vi "check_point_inside_rect.vi"(5 "rectangle corner":dbl[][](array[numeric]), 8 "Y":dbl[](array[numeric]), 11 "X":dbl[](array[numeric])) -> (3 "result":bool)   [LabVIEW 2017]
panel:
  out "py":dbl
  out "px":dbl
  out "p4y":dbl
  out "p4x":dbl
  out "p3y":dbl
  out "p3x":dbl
  out "p2y":dbl
  out "p2x":dbl
  out "p1y":dbl
  out "p1x":dbl
  out "length condition":bool
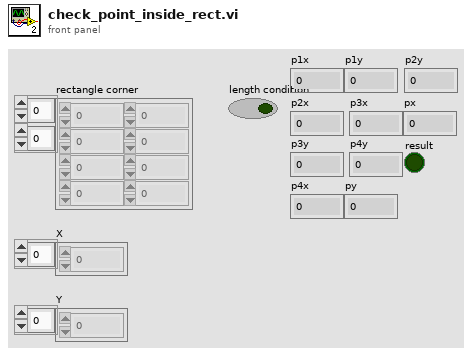
[diagram p1: front panel]
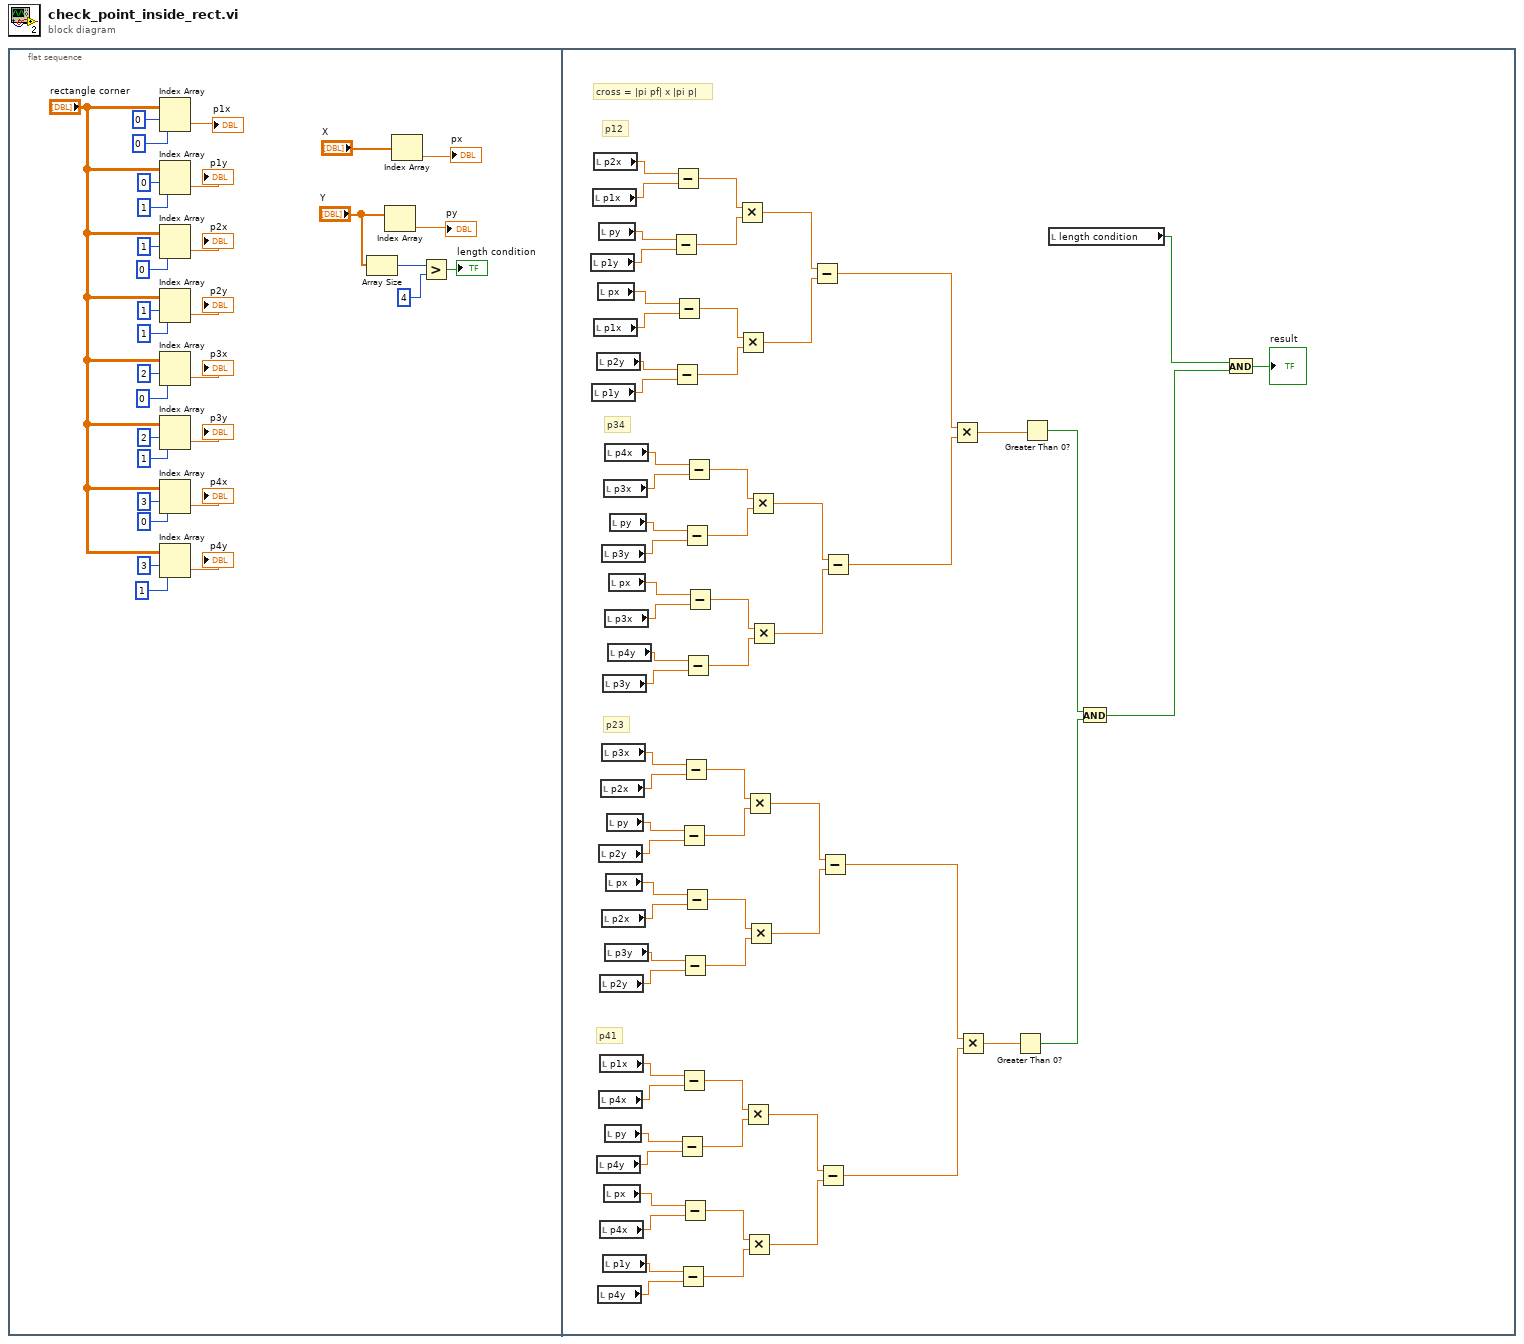
[diagram p0: block diagram]
diagram:
  n1 = flat-sequence {
    frame #0 {
      n2 = Index Array(array="rectangle corner", index (row)=0, index (col)=0 ("disabled index (col)")) -> (element=→"p1x":dbl)
      n3 = Index Array(array="rectangle corner", index (row)=0, index (col)=1 ("disabled index (col)")) -> (element=→"p1y":dbl)
      n4 = Index Array(array="rectangle corner", index (row)=1, index (col)=0 ("disabled index (col)")) -> (element=→"p2x":dbl)
      n5 = Index Array(array="rectangle corner", index (row)=1, index (col)=1 ("disabled index (col)")) -> (element=→"p2y":dbl)
      n6 = Index Array(array="rectangle corner", index (row)=2, index (col)=0 ("disabled index (col)")) -> (element=→"p3x":dbl)
      n7 = Index Array(array="rectangle corner", index (row)=2, index (col)=1 ("disabled index (col)")) -> (element=→"p3y":dbl)
      n8 = Index Array(array="rectangle corner", index (row)=3, index (col)=0 ("disabled index (col)")) -> (element=→"p4x":dbl)
      n9 = Index Array(array="rectangle corner", index (row)=3, index (col)=1 ("disabled index (col)")) -> (element=→"p4y":dbl)
      n10 = Array Size(array="Y") -> (size(s)=w4:i32)
      n11 = Index Array(array="Y") -> (element=→"py":dbl)  [unwired: 1 in]
      n12 = Index Array(array="X") -> (element=→"px":dbl)  [unwired: 1 in]
      n13 = Greater?(x=w4, y=4) -> (0:→"length condition":bool)
    }
    frame #1 {
      # "p41"
      # "p34"
      # "p23"
      # "cross = |pi pf| x |pi p|"
      # "p12"
      n14 = local read "p1y"() -> (w96:dbl)
      n15 = local read "p1y"() -> (w91:dbl)
      n16 = local read "p1x"() -> (w98:dbl)
      n17 = local read "p2x"() -> (w99:dbl)
      n18 = local read "p1x"() -> (w89:dbl)
      n19 = local read "p2y"() -> (w90:dbl)
      n20 = local read "p4y"() -> (w47:dbl)
      n21 = local read "px"() -> (w88:dbl)
      n22 = local read "p4y"() -> (w52:dbl)
      n23 = local read "py"() -> (w97:dbl)
      n24 = local read "p2y"() -> (w75:dbl)
      n25 = local read "p4x"() -> (w45:dbl)
      n26 = local read "p2y"() -> (w80:dbl)
      n27 = local read "p1x"() -> (w44:dbl)
      n28 = local read "p4x"() -> (w54:dbl)
      n29 = local read "p2x"() -> (w73:dbl)
      n30 = local read "p3y"() -> (w68:dbl)
      n31 = local read "p3x"() -> (w72:dbl)
      n32 = local read "p2x"() -> (w82:dbl)
      n33 = local read "p3y"() -> (w63:dbl)
      n34 = local read "p1y"() -> (w53:dbl)
      n35 = local read "p3x"() -> (w70:dbl)
      n36 = local read "px"() -> (w55:dbl)
      n37 = local read "p4x"() -> (w71:dbl)
      n38 = local read "p3x"() -> (w61:dbl)
      n39 = local read "p3y"() -> (w81:dbl)
      n40 = local read "py"() -> (w46:dbl)
      n41 = local read "px"() -> (w83:dbl)
      n42 = local read "py"() -> (w74:dbl)
      n43 = local read "p4y"() -> (w62:dbl)
      n44 = local read "px"() -> (w60:dbl)
      n45 = local read "py"() -> (w69:dbl)
      n46 = Subtract(x=w97, y=w96) -> (x-y=w94:dbl)
      n47 = Subtract(x=w90, y=w91) -> (x-y=w93:dbl)
      n48 = Subtract(x=w99, y=w98) -> (x-y=w95:dbl)
      n49 = Subtract(x=w88, y=w89) -> (x-y=w92:dbl)
      n50 = Subtract(x=w46, y=w47) -> (x-y=w49:dbl)
      n51 = Subtract(x=w53, y=w52) -> (x-y=w50:dbl)
      n52 = Subtract(x=w74, y=w75) -> (x-y=w77:dbl)
      n53 = Subtract(x=w44, y=w45) -> (x-y=w48:dbl)
      n54 = Subtract(x=w81, y=w80) -> (x-y=w78:dbl)
      n55 = Subtract(x=w55, y=w54) -> (x-y=w51:dbl)
      n56 = Subtract(x=w72, y=w73) -> (x-y=w76:dbl)
      n57 = Subtract(x=w69, y=w68) -> (x-y=w66:dbl)
      n58 = Subtract(x=w83, y=w82) -> (x-y=w79:dbl)
      n59 = Subtract(x=w62, y=w63) -> (x-y=w65:dbl)
      n60 = Subtract(x=w71, y=w70) -> (x-y=w67:dbl)
      n61 = Subtract(x=w60, y=w61) -> (x-y=w64:dbl)
      n62 = Multiply(x=w95, y=w94) -> (x*y=w87:dbl)
      n63 = Multiply(x=w92, y=w93) -> (x*y=w86:dbl)
      n64 = Multiply(x=w48, y=w49) -> (x*y=w56:dbl)
      n65 = Multiply(x=w51, y=w50) -> (x*y=w57:dbl)
      n66 = Multiply(x=w76, y=w77) -> (x*y=w84:dbl)
      n67 = Multiply(x=w79, y=w78) -> (x*y=w85:dbl)
      n68 = Multiply(x=w67, y=w66) -> (x*y=w59:dbl)
      n69 = Multiply(x=w64, y=w65) -> (x*y=w58:dbl)
      n70 = Subtract(x=w87, y=w86) -> (x-y=w43:dbl)
      n71 = Subtract(x=w56, y=w57) -> (x-y=w39:dbl)
      n72 = Subtract(x=w84, y=w85) -> (x-y=w40:dbl)
      n73 = Subtract(x=w59, y=w58) -> (x-y=w42:dbl)
      n74 = Multiply(x=w43, y=w42) -> (x*y=w41:dbl)
      n75 = Multiply(x=w40, y=w39) -> (x*y=w38:dbl)
      n76 = Greater Than 0?(x=w38) -> (x > 0?=w36:bool)
      n77 = Greater Than 0?(x=w41) -> (x > 0?=w37:bool)
      n78 = local read "length condition"() -> (w35:bool)
      n79 = And(x=w37, y=w36) -> (x .and. y?=w34:bool)
      n80 = And(x=w35, y=w34) -> (x .and. y?=→"result":bool)
    }
  }
